vi "加标回收启动 (子VI).vi"(11 "启动参数":T1(ring)=enum."CODCr") -> (0 "error out":T2={"status"=FALSE, "代码"=4, "source"=""} caption="错误输出" {"代码" items=["执行成功"=1, "执行失败，但不知道原因"=2, "命令请求条件错误"=3, "通讯超时"=4, "系统繁忙不能执行"=5, "系统故障"=6, "没有数据"=100]})   [LabVIEW 2016, in "MB SLAVE.lvlib"]
uses:
  MB SLAVE.lvlib
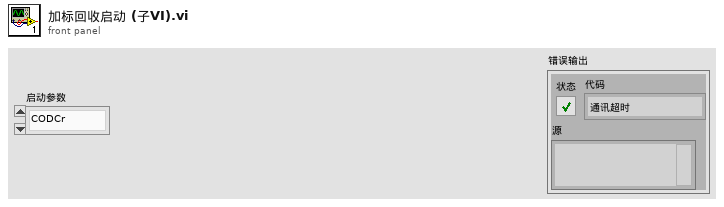
[diagram p1: front panel]
types:
  T1 = enum16{"未选择", "CODMn", "氨氮", "总磷", "总氮", "CODCr"}
  T2 = cluster{"status":bool, "代码":u16, "source":string}
  T3 = typedef "质控单元V4.lvlib/测试子流程.ctl" = enum16{"水样测试（润洗采样分开）", "水样测试（润洗采样合并）", "水样测试（不启动采配水）", "加标回收（润洗采样分开）", "加标回收（润洗采样合并）", "加标回收（不启动采配水）", "集成干预测试", "平行样测试", "平行样测试（不启动采配水）", "水样测试（不含采样杯）", "平行样测试（不含采样杯）", "集成干预测试（不含采样杯）"}
  T4 = typedef "质控单元V4.lvlib/质控slave id.ctl" = enum16{"null", "氨氮", "总磷", "总氮", "CODMn", "CODCr", "氟化物"}
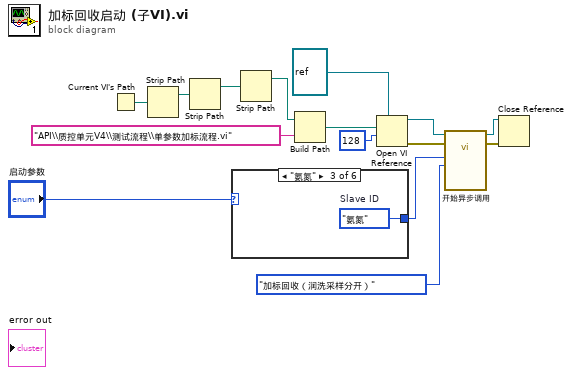
[diagram p0: block diagram]
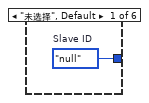
[diagram p2: hidden frame]
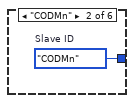
[diagram p3: hidden frame]
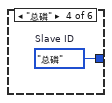
[diagram p4: hidden frame]
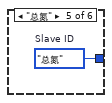
[diagram p5: hidden frame]
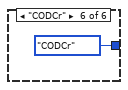
[diagram p6: hidden frame]
diagram:
  n1 = Current VI's Path() -> (path=w14:path)
  n2 = Strip Path(path=w14) -> (stripped path=w3:path)  [unwired: 1 out]
  n3 = Strip Path(path=w3) -> (stripped path=w2:path)  [unwired: 1 out]
  n4 = case shown="\"氨氮\"" "启动参数" {
    tunnel: [w16 w17 w18 w19 w20 质控slave_id."CODCr" ("Slave ID")] -> w1
    frame "未选择", Default {
      w16 = 质控slave_id."null"  # Slave ID
    }
    frame "CODMn" {
      w17 = 质控slave_id."CODMn"  # Slave ID
    }
    frame "氨氮" {
      w18 = 质控slave_id."氨氮"  # Slave ID
    }
    frame "总磷" {
      w19 = 质控slave_id."总磷"  # Slave ID
    }
    frame "总氮" {
      w20 = 质控slave_id."总氮"  # Slave ID
    }
    frame "CODCr" {
    }
  }
  n5 = Strip Path(path=w2) -> (stripped path=w12:path)  [unwired: 1 out]
  n6 = Build Path(base path=w12, name or relative path="API\\质控单元V4\\测试流程\\单参数加标流程.vi" ("名称或相对路径")) -> (appended path=w5:path)
  n7 = Open VI Reference(type specifier VI Refnum (for type only)=refnum<vi> refnum, vi path=w5, options=128 ("选项")) -> (vi reference=w8:refnum<vi>, error out=w9:errorcluster)  [unwired: 3 in]
  n8 = call-by-ref "开始异步调用"(reference=w8, error in=w9, "流程类型"=测试子流程."加标回收（润洗采样分开）", "Slave ID"=w1) -> (reference out=w10:refnum<vi>, error out=w11:errorcluster)  [unwired: 10 in]
  n9 = Close Reference(reference=w10, error in (no error)=w11) -> ()  [unwired: 1 out]
